vi "propertyConfigs.set.vi"(8 "error in (no error)":errorcluster, 10 "properties":T1, 11 "type in":refnum<class "type.lvclass">) -> (0 "error out":errorcluster, 3 "type out":refnum<class "type.lvclass">)   [LabVIEW 2020, in "type.lvclass"]
uses:
  type.lvclass
  properties.ctl
  property.ctl
  property value.ctl
  type.lvclass/type.ctl
  Nominal Client/Nominal Client.lvclass/Nominal Client.ctl
  Nominal Client/error.vi
  Nominal Client/trace.payload_sent.vi
  Nominal Client/trace.payload_received.vi
  Nominal Client/create.authorization_header.vi
  Nominal Client/error.vi/859f8e04-e495-489b-b5b4-7ac163f56130.vi
  Nominal Client/trace.generate.vi
  <vilib>/AdvancedString/1D String Array to Delimited String.vi
  <vilib>/JDP Science/JDP Science Common Utilities/Trim Whitespace__JDP.vi
  Nominal Client/trace.calling_method.vi
  Nominal Client/api_token.get.vi
  <vilib>/JDP Science/JSONtext/support/Format JSON Object.vi
  <vilib>/Utility/libraryn.llb/Get File Extension.vi
  Nominal Client/log_file.write.vi
  <vilib>/JDP Science/JSONtext/Get all Object Items.vi
  <vilib>/Utility/error.llb/Error Cluster From Error Code.vi
  <vilib>/JDP Science/JSONtext/JSON text to Variant.vi
  <vilib>/JDP Science/JSONtext/LVClass Serializer/JSONtext LVClass Serializer.lvclass
  <vilib>/addons/_JKI.lib/REST Client/classes/Response Headers/Response Headers.lvclass
  <vilib>/addons/_JKI.lib/REST Client/classes/REST Client/REST Client.lvclass
  Nominal Client/Nominal Client.lvclass
  <vilib>/JDP Science/JSONtext/JSONtext.lvlib
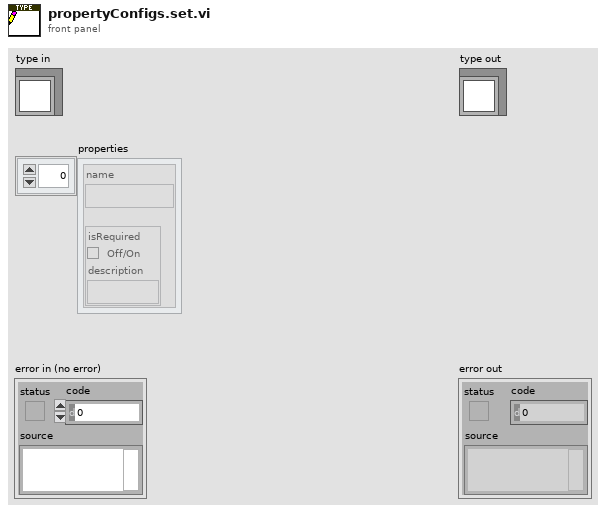
[diagram p1: front panel]
types:
  T1 = typedef "type.lvclass/properties.ctl" = T2[]
  T2 = typedef "type.lvclass/property.ctl" = cluster{"name":string, "value":T3}
  T3 = typedef "type.lvclass/property value.ctl" = cluster{"isRequired":bool, "description":string}
  T4 = typedef "type.lvclass/typeData.ctl" = cluster{"rid":string, "name":string, "description":string, "propertyConfigs":T1, "createdAt":timestamp, "datasourceConfigs":T5[], "iconName":string}
  T5 = typedef "type.lvclass/datasourceConfig.ctl" = cluster{"name":string, "v1":string[], "suggestedRefName":string}
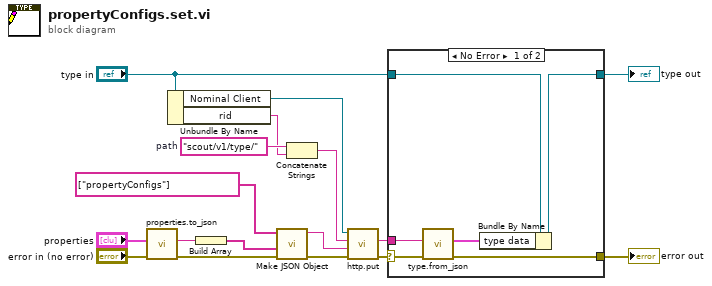
[diagram p0: block diagram]
diagram:
  w15 = "scout/v1/type/"  # path
  n1 = call "properties.to_json.vi"("error in"="error in (no error)", "properties"="properties") -> ("error out"=w3:errorcluster, "json"=w5:string)  [unwired: 8 in]
  n2 = Unbundle By Name("type in") -> ("Nominal Client"=w16:refnum<class "Nominal Client.lvclass">, "rid"=w13:string)
  n3 = Build Array(w5) -> (w4:string[])
  n4 = call <vilib>:"Make JSON Object.vi"("error in (no error)"=w3, "JSON Items"=w4, "Item Names"=string[] ["propertyConfigs"]) -> ("error out"=w2:errorcluster, "<JSON>"=w1:string)  [unwired: 7 in]
  n5 = Concatenate Strings(w15, w13) -> (w14:string)
  n6 = call "http.put.vi"("error in"=w2, "Body"=w1, "Path"=w14, "Nominal Client in"=w16) -> ("error out"=w12:errorcluster, "Response"=w11:string)  [unwired: 4 in, 2 out]
  n7 = case shown="No Error" w12 {
    selector: w12 -> [w21 w25]
    tunnel: [w20 w25] -> w8
    tunnel: "type in" -> [w23 w24]
    tunnel: w11 -> [w19 _]
    tunnel: [w22 w24] -> w9
    frame No Error {
      n8 = call "type.from_json.vi"("error in"=w21, "json"=w19) -> ("error out"=w20:errorcluster, "type data"=w18:T4)  [unwired: 8 in]
      n9 = Bundle By Name(cluster=w23, "type data"=w18) -> (w22:refnum<class "type.lvclass">)
    }
    frame Error {
    }
  }
  "error out" <- w8
  "type out" <- w9
